vi "分段显示曲线的绘制.vi"() -> ()   [LabVIEW 2014]
panel:
  out "分段显示曲线":dbl[][](graph) caption="分段显示波形图"
  out "元素索引":i32
  out "中断的曲线":dbl[](graph) caption="波形图"
  out "数组":dbl[](array[numeric])
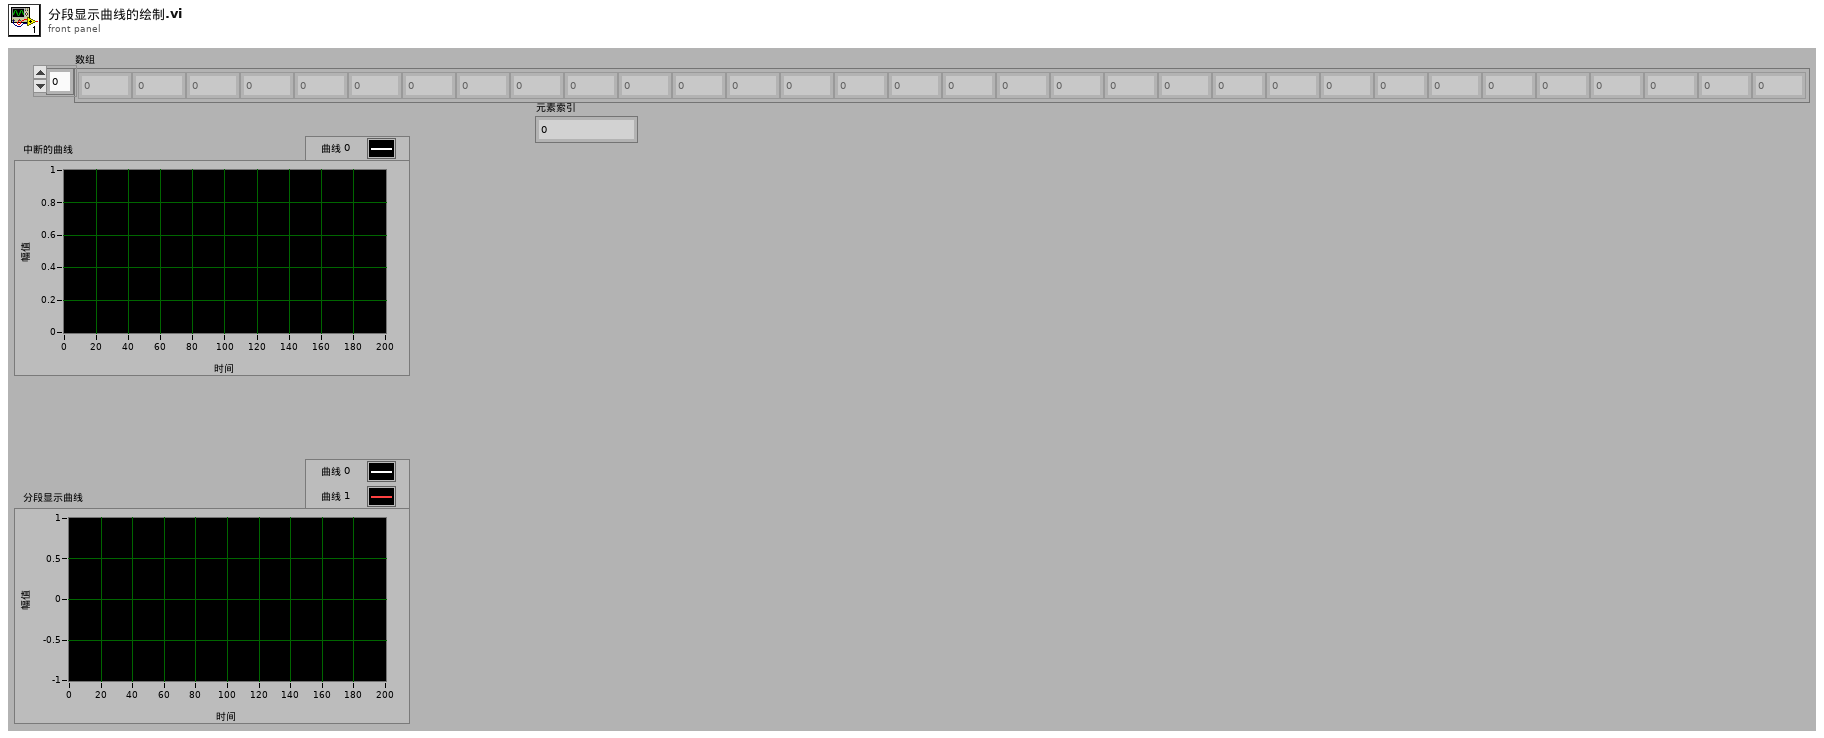
[diagram p1: front panel]
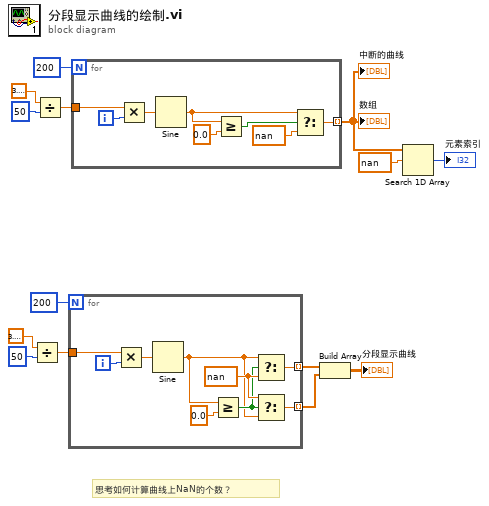
[diagram p0: block diagram]
diagram:
  # "思考如何计算曲线上NaN的个数？"
  n1 = Divide(x=3.141592653589793, y=50) -> (x/y=w6:dbl)
  n2 = Divide(x=3.141592653589793, y=50) -> (x/y=w12:dbl)
  n3 = for {
    N: 200 -> [_]
    tunnel: w6 -> [w23]
    tunnel: [w19] -> w3 mode=indexing
    tunnel: [w15] -> w2 mode=indexing
    i -> [w22]
    w18 = nan ("y")
    n4 = Multiply(x=w23, y=w22) -> (x*y=w21:dbl)
    n5 = Sine(x=w21) -> (sin(x)=w16:dbl)
    n6 = Greater Or Equal?(x=w16, y=0.0) -> (x >= y?=w17:bool)
    n7 = Select(t=w16, s=w17, f=w18) -> (s? t:f=w19:dbl)
    n8 = Select(t=w18, s=w17, f=w16) -> (s? t:f=w15:dbl)
  }
  n9 = for {
    N: 200 -> [_]
    tunnel: w12 -> [w31]
    tunnel: [w24] -> w8 mode=indexing
    i -> [w30]
    n10 = Multiply(x=w31, y=w30) -> (x*y=w29:dbl)
    n11 = Sine(x=w29) -> (sin(x)=w26:dbl)
    n12 = Greater Or Equal?(x=w26, y=0.0) -> (x >= y?=w27:bool)
    n13 = Select(t=w26, s=w27, f=nan ("y")) -> (s? t:f=w24:dbl)
  }
  "数组" <- w8
  "中断的曲线" <- w8
  n14 = Build Array(w3, w2) -> (→"分段显示曲线":dbl[][])
  n15 = Search 1D Array(1D array=w8, element=nan ("y")) -> (index of element=→"元素索引":i32)  [unwired: 1 in]
